vi "Determine Warnings V2.vi"() -> ()   [LabVIEW 2014]
panel:
  out "warning?":bool
  out "warning text":string
  in  "min temp":dbl
  in  "max temp":dbl
  in  "current temp":dbl
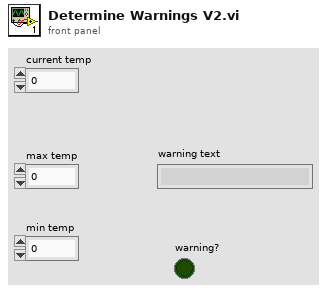
[diagram p1: front panel]
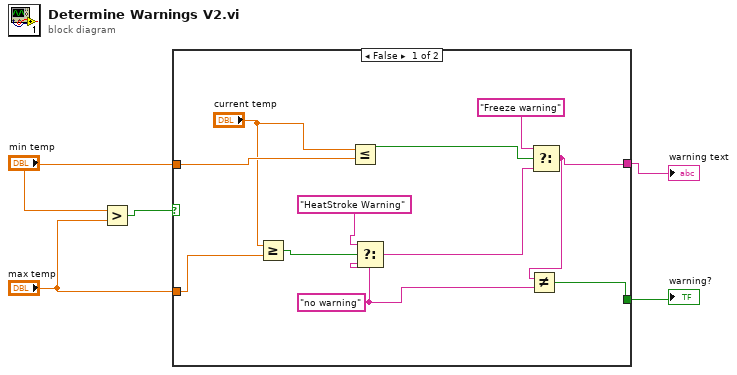
[diagram p0: block diagram]
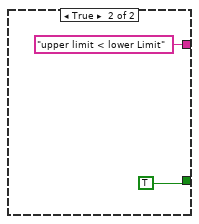
[diagram p2: hidden frame]
diagram:
  n1 = Greater?(x="min temp", y="max temp") -> (0:w3:bool)
  n2 = case shown="False" w3 {
    tunnel: "min temp" -> [w16 _]
    tunnel: "max temp" -> [w11 _]
    tunnel: [w8 "upper limit < lower Limit"] -> w2
    tunnel: [w6 TRUE] -> w1
    frame False {
      w7 = "no warning"
      n3 = Greater Or Equal?(x="current temp", y=w11) -> (x >= y?=w9:bool)
      n4 = Less Or Equal?(x="current temp", y=w16) -> (x <= y?=w15:bool)
      n5 = Select(t="HeatStroke Warning", s=w9, f=w7) -> (s? t:f=w12:string)
      n6 = Select(t="Freeze warning", s=w15, f=w12) -> (s? t:f=w8:string)
      n7 = Not Equal?(x=w8, y=w7) -> (x != y?=w6:bool)
    }
    frame True {
    }
  }
  "warning text" <- w2
  "warning?" <- w1
